vi "Read.vi"(8 "error in (no error)":errorcluster, 11 "TroSpec in":refnum<class "PL ISTEQ TroSpec.lvclass">) -> (0 "error out":errorcluster, 2 "data":u8[](array[numeric]), 3 "TroSpec out":refnum<class "PL ISTEQ TroSpec.lvclass">)   [LabVIEW 2015, in "PL ISTEQ TroSpec.lvclass"]
doc: "Reads data from the device."
uses:
  PL ISTEQ TroSpec.lvclass
  PL ISTEQ TroSpec.lvclass/PL ISTEQ TroSpec.ctl
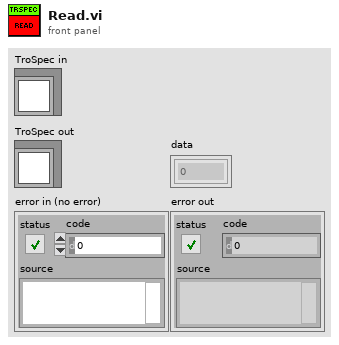
[diagram p1: front panel]
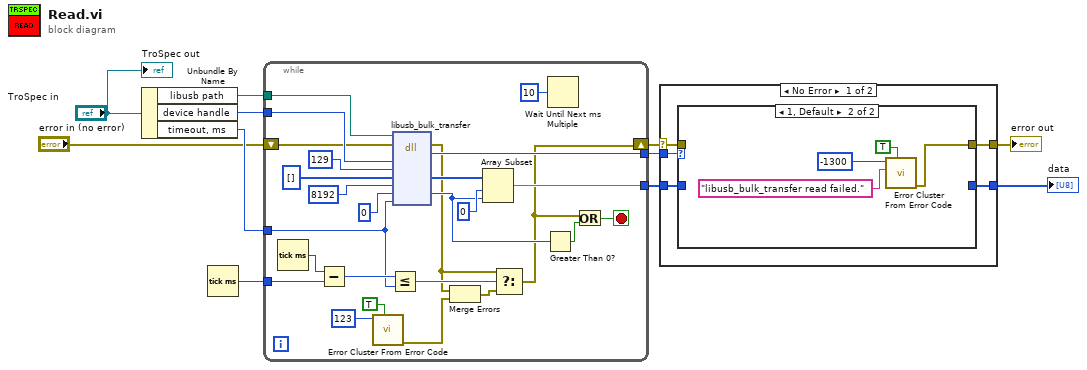
[diagram p0: block diagram]
diagram:
  n1 = Unbundle By Name("TroSpec in") -> ("libusb path"=w11:path, "device handle"=w10:u64, "timeout, ms"=w9:u32)
  n2 = Tick Count (ms)() -> (millisecond timer value=w1:u32)
  n3 = while {
    tunnel: w11 -> [w37]
    tunnel: w10 -> [w36]
    tunnel: w9 -> [w22]
    tunnel: [w34] -> w7
    tunnel: [w28] -> w2
    shift-right: [w15] -> w8
    shift-left: "error in (no error)" -> [w33]
    tunnel: w1 -> [w24]
    stop <- w19 stop-if-true
    n4 = Tick Count (ms)() -> (millisecond timer value=w25:u32)
    n5 = Subtract(x=w25, y=w24) -> (x-y=w23:u32)
    n6 = call <vilib>:"Error Cluster From Error Code.vi"("show call chain? (False)"=TRUE, "error code (0)"=123) -> ("error out"=w14:errorcluster)  [unwired: 7 in]
    n7 = Less Or Equal?(x=w23, y=w22) -> (x <= y?=w16:bool)
    n8 = dll-call lib="D:/Temp/libusb/libusb-1.0-x64.dll" fn="libusb_bulk_transfer"(path in=w37, error in=w33, "dev_handle"=w36, "endpoint"=u8 129 ("bmRequestType"), "data"=u8[] [], "length"=8192, "transferred"=0, "timeout"=w22) -> (error out=w12:errorcluster, "return type"=w34:i32, "data"=w29:u8[], "transferred"=w21:i32)  [unwired: 5 in, 1 out]
    n9 = Merge Errors(w12, w14) -> (w13:errorcluster)
    n10 = Array Subset(array=w29, index=0, length=w21) -> (w28:u8[])
    n11 = Select(t=w12, s=w16, f=w13) -> (s? t:f=w15:errorcluster)
    n12 = Greater Than 0?(x=w21) -> (x > 0?=w20:bool)
    n13 = Wait Until Next ms Multiple(millisecond multiple=u32 10) -> ()  [unwired: 1 out]
    n14 = Or(x=w15, y=w20) -> (x .or. y?=w19:bool)
  }
  n15 = case shown="No Error" w8 {
    selector: w8 -> [w41 w49]
    tunnel: w7 -> [w42 _]
    tunnel: [w40 w49] -> w5
    tunnel: w2 -> [w39 _]
    tunnel: [w38 _] -> w3
    frame No Error {
      n16 = case shown="1, Default" w42 {
        tunnel: w41 -> [w44 _]
        tunnel: [w44 w45] -> w40
        tunnel: w39 -> [w43 _]
        tunnel: [w43 _] -> w38
        frame 0 {
        }
        frame 1, Default {
          n17 = call <vilib>:"Error Cluster From Error Code.vi"("show call chain? (False)"=TRUE, "error message (\"\")"="libusb_bulk_transfer read failed." ("format string"), "error code (0)"=-1300) -> ("error out"=w45:errorcluster)  [unwired: 6 in]
        }
      }
    }
    frame Error {
    }
  }
  "error out" <- w5
  "data" <- w3
  "TroSpec out" <- "TroSpec in"
